vi "skippable_AlliGator SS1 Dataset Laser Frequency Dialog.vi"(8 "Error In":errorcluster) -> (0 "Error Out":errorcluster, 3 "Laser Frequency":dbl[unit] format="%#g")   [LabVIEW 2021, in "AlliGator Files.lvlib"]
doc: "Dialog to ask the user for the laser frequency used to record the dataset. This is different from the detector trigger frequency, which is always close to 20 MHz."
uses:
  AlliGator/AlliGator Files.lvlib
  <vilib>/Utility/error.llb/Error Cluster From Error Code.vi
  <vilib>/ErrorRing/Error Ring.xnode
  AlliGator/AlliGator GUI.lvlib
  Sound/Sound.lvlib
panel:
  in  "Laser Frequency":dbl[unit]=80000000.0 min=0.0 format="%#g"
  in  "Cancel":bool
  in  "OK":bool
  in  "Do not show this dialog again":bool
  out "Displayed Message":string="Specify the laser frequency used during acquisition:"
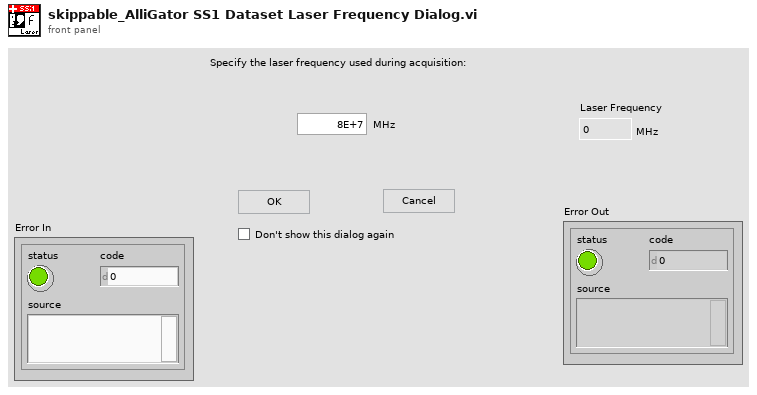
[diagram p1: front panel]
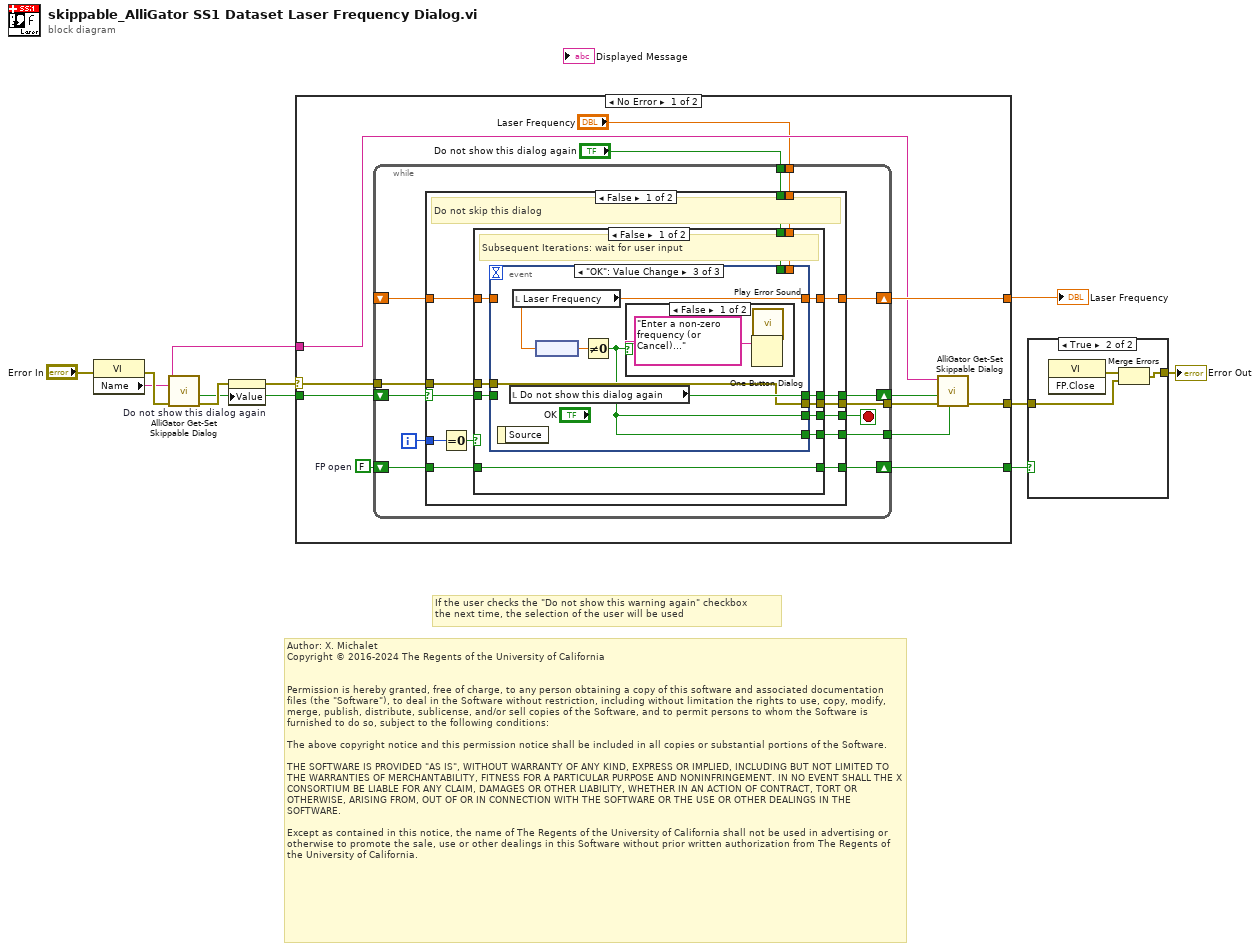
[diagram p0: block diagram]
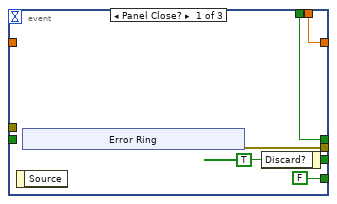
[diagram p3: hidden frame]
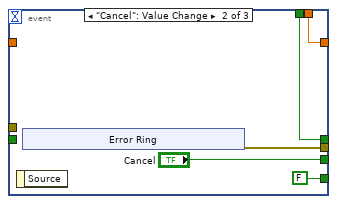
[diagram p4: hidden frame]
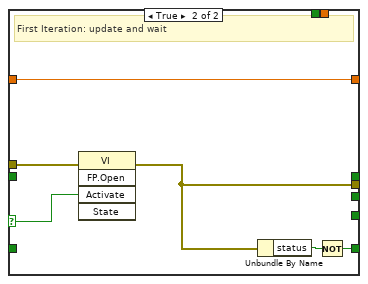
[diagram p6: hidden frame]
diagram:
  # "Author: X. Michalet\nCopyright © 2016-2024 The Regents of the University of California\n \n\nPermission is hereby granted, free of charge, to any person obtaining a copy of this software and associated documentation files (the \"Software\"), to deal in the Software without restriction, including without limitation the rights to use, copy, modify, merge, publish, distribute, sublicense, and/or sell copies of the Software, and to permit persons to whom the Software is furnished to do so, subject to the following conditions:\n\nThe above copyright notice and this permission notice shall be included in all copies or substantial portions of the Software.\n\nTHE SOFTWARE IS PROVIDED \"AS IS\", WITHOUT WARRANTY OF ANY KIND, EXPRESS OR IMPLIED, INCLUDING BUT NOT LIMITED TO THE WARRANTIES OF MERCHANTABILITY, FITNESS FOR A PARTICULAR PURPOSE AND NONINFRINGEMENT. IN NO EVENT SHALL THE X CONSORTIUM BE LIABLE FOR ANY CLAIM, DAMAGES OR OTHER LIABILITY, WHETHER IN AN ACTION OF CONTRACT, TORT OR OTHERWISE, ARISING FROM, OUT OF OR IN CONNECTION WITH THE SOFTWARE OR THE USE OR OTHER DEALINGS IN THE SOFTWARE.\n\nExcept as contained in this notice, the name of The Regents of the University of California shall not be used in advertising or otherwise to promote the sale, use or other dealings in this Software without prior written authorization from The Regents of the University of California."
  # "If the user checks the \"Do not show this warning again\" checkbox\nthe next time, the selection of the user will be used"
  n1 = property class="VI"(error in="Error In") -> (error out=w9:errorcluster, "Name"=w8:string)  [unwired: 1 in, 1 out]
  n2 = call "AlliGator Get-Set Skippable Dialog.vi"("Error In"=w9, "Dialog Window VI Name"=w8) -> ("Error Out"=w5:errorcluster, "Is skipped (out)"=w4:bool)  [unwired: 8 in]
  n3 = property on="Do not show this dialog again" class="Bool (strict)"(error in=w5, "Value"=w4) -> (error out=w3:errorcluster)  [unwired: 1 in, 1 out]
  n4 = case shown="No Error" w3 {
    selector: w3 -> [w15 w95]
    tunnel: [w22 _] -> w2
    tunnel: w4 -> [w21 _]
    tunnel: w8 -> [w18 _]
    tunnel: [w17 w95] -> w7
    tunnel: [w11 _] -> w1
    frame No Error {
      w12 = FALSE  # FP open
      n5 = while {
        shift-right: [w35] -> w19
        shift-left: w21 -> [w33]
        shift-right: [w30] -> w22
        shift-left: _ -> [w31]
        tunnel: "Do not show this dialog again" -> [w29]
        tunnel: [w28] -> w16
        tunnel: "Laser Frequency" -> [w27]
        tunnel: w15 -> [w26]
        tunnel: [w25] -> w14
        shift-right: [w23] -> w11
        shift-left: w12 -> [w24]
        i -> [w34]
        stop <- w32 stop-if-true
        n6 = case shown="False" w33 {
          selector: w33 -> [w47 w93]
          tunnel: [w49 w93] -> w35
          tunnel: w34 -> [w48 _]
          tunnel: [w46 w93] -> w32
          tunnel: w31 -> [w45 w94]
          tunnel: [w44 w94] -> w30
          tunnel: w29 -> [w43 _]
          tunnel: [w41 w93] -> w28
          tunnel: w27 -> [w40 _]
          tunnel: w26 -> [w39 w92]
          tunnel: [w38 w92] -> w25
          tunnel: w24 -> [w37 w91]
          tunnel: [w36 w91] -> w23
          frame False {
            # "Do not skip this dialog"
            n7 = Equal To 0?(x=w48) -> (x = 0?=w42:bool)
            n8 = case shown="False" w42 {
              selector: w42 -> [_ w90]
              tunnel: [w60 _] -> w46
              tunnel: [w59 _] -> w49
              tunnel: w47 -> [w58 _]
              tunnel: w45 -> [w57 w89]
              tunnel: [w56 w89] -> w44
              tunnel: w43 -> [w55 _]
              tunnel: [w54 _] -> w41
              tunnel: w40 -> [w53 _]
              tunnel: w39 -> [w52 w88]
              tunnel: [w51 w87] -> w38
              tunnel: w37 -> [w50 _]
              tunnel: [w50 w85] -> w36
              frame False {
                # "Subsequent Iterations: wait for user input"
                n9 = event shown="[2] \"OK\": Value Change" {
                  selector: _ -> [_ _ _]
                  dyn-events: _ -> [_ _ _]
                  timeout: _ -> [_ _ _]
                  tunnel: [w65 "Cancel" w79] -> w60
                  tunnel: [w64 w74 w83] -> w59
                  tunnel: w58 -> [_ _ _]
                  tunnel: w57 -> [_ _ _]
                  tunnel: [w62 w72 w81] -> w56
                  tunnel: w55 -> [w64 w74 _]
                  tunnel: [FALSE ("Discard?") FALSE ("Discard?") w79] -> w54
                  tunnel: w53 -> [w62 w72 _]
                  tunnel: w52 -> [_ _ w82]
                  tunnel: [w61 w71 w82] -> w51
                  event Panel Close? {
                    w65 = TRUE ("Discard?")
                    n10 = event-data() -> ()  [unwired: 1 in, 1 out]
                    n11 = xnode "Error Ring"() -> ("error out"=w61:errorcluster)
                    n12 = event-data("Discard?"=w65) -> ()  [unwired: 1 in, 1 out]
                  }
                  event "Cancel": Value Change {
                    n13 = event-data() -> ()  [unwired: 1 in, 1 out]
                    n14 = xnode "Error Ring"() -> ("error out"=w71:errorcluster)
                  }
                  event "OK": Value Change {
                    n15 = event-data() -> ()  [unwired: 1 in, 1 out]
                    n16 = local read "Do not show this dialog again"() -> (w83:bool)
                    n17 = local read "Laser Frequency"() -> (w81:dbl[unit])
                    n18 = node(w81) -> (w80:dbl)
                    n19 = Not Equal To 0?(x=w80) -> (x != 0?=w79:bool)
                    n20 = case shown="False" w79 {
                      frame False {
                        n21 = One Button Dialog(message="Enter a non-zero frequency (or Cancel)...") -> ()  [unwired: 1 in, 1 out]
                        n22 = call "Play Error Sound.vi"() -> ()  [unwired: 27 in, 1 out]
                      }
                      frame True {
                      }
                    }
                  }
                }
              }
              frame True {
                # "First Iteration: update and wait"
                n23 = invoke class="VI" method="FP.Open"(error in=w88, "Activate"=w90) -> (error out=w87:errorcluster)  [unwired: 3 in, 4 out]
                n24 = Unbundle By Name(w87) -> ("status"=w86:bool)
                n25 = Not(x=w86) -> (.not. x?=w85:bool)
              }
            }
          }
          frame True {
            # "skip this dialog"
          }
        }
      }
      n26 = call "AlliGator Get-Set Skippable Dialog.vi"("Set/Get (F)"=w16, "Error In"=w14, "Is skipped (in)"=w19, "Dialog Window VI Name"=w18) -> ("Error Out"=w17:errorcluster)  [unwired: 6 in, 1 out]
    }
    frame Error {
    }
  }
  "Laser Frequency" <- w2
  n27 = case shown="True" w1 {
    tunnel: w7 -> [w96 w97]
    tunnel: [w96 w98] -> w6
    frame False {
    }
    frame True {
      n28 = invoke class="VI" method="FP.Close"() -> (error out=w99:errorcluster)  [unwired: 3 in, 2 out]
      n29 = Merge Errors(w99, w97) -> (w98:errorcluster)
    }
  }
  "Error Out" <- w6
